vi "Facade.vi"(0 "Data In":T4, 2 "Display State In":T2, 3 "Container State":T3) -> (6 "Data Out":T4, 7 "Display State Out":T2, 8 "Action":T1)   [LabVIEW 2020, in "AM.xctl"]
uses:
  AM.xctl
  Data.vi
  Classes/Modulations/AM/AM.lvclass
  D:/Development/epl-vi-lib/Koop/KObject Class/KObject.lvclass
  <vilib>/_xctls/Container State.ctl
  State.vi
  <vilib>/_xctls/Action.ctl
  SAM/SAM.xctl
  Classes/Modulations/SAM/SAM.lvclass
  D:/Development/epl-vi-lib/Signal Synthesis VIs/4th Generation/Classes/Modulations/AM/AM.lvclass
  Classes/Modulations/AM/AM.lvclass/AM.ctl
  Classes/Modulations/AM/Write Depth (0-1).vi
  Classes/Modulations/AM/Write Correct level .vi
  Classes/Modulations/AM/Read Depth (0-1).vi
  Classes/Modulations/AM/Read Correct level .vi
  <vilib>/_xctls/XControlSupport.lvlib
  Koop/KObject Class/KObject.lvclass
panel:
  in  "Apply level correction":bool
  in  "Depth (0-1)":dbl min=0.0 max=1.0
  in  "Tabs":enum32{"OFF", "SAM"}(tab)
  in  "SAM":refnum<class "SAM.lvclass">(xcontrol)
  in  "Shape":u16(ring) items=["OFF", "SAM"]
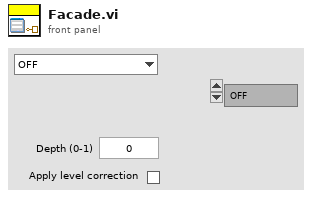
[diagram p1: front panel]
types:
  T1 = typedef "XControlSupport.lvlib/Action.ctl" = cluster{"Data Changed?":bool, "State Changed?":bool, "Action Name":string}
  T2 = typedef "AM.xctl/State.vi" = cluster{"Numeric":dbl}
  T3 = typedef "XControlSupport.lvlib/Container State.ctl" = cluster{"Indicator?":bool, "Run Mode?":bool, " Refnum":refnum<vi>}
  T4 = typedef "AM.xctl/Data.vi" = refnum<class "AM.lvclass">
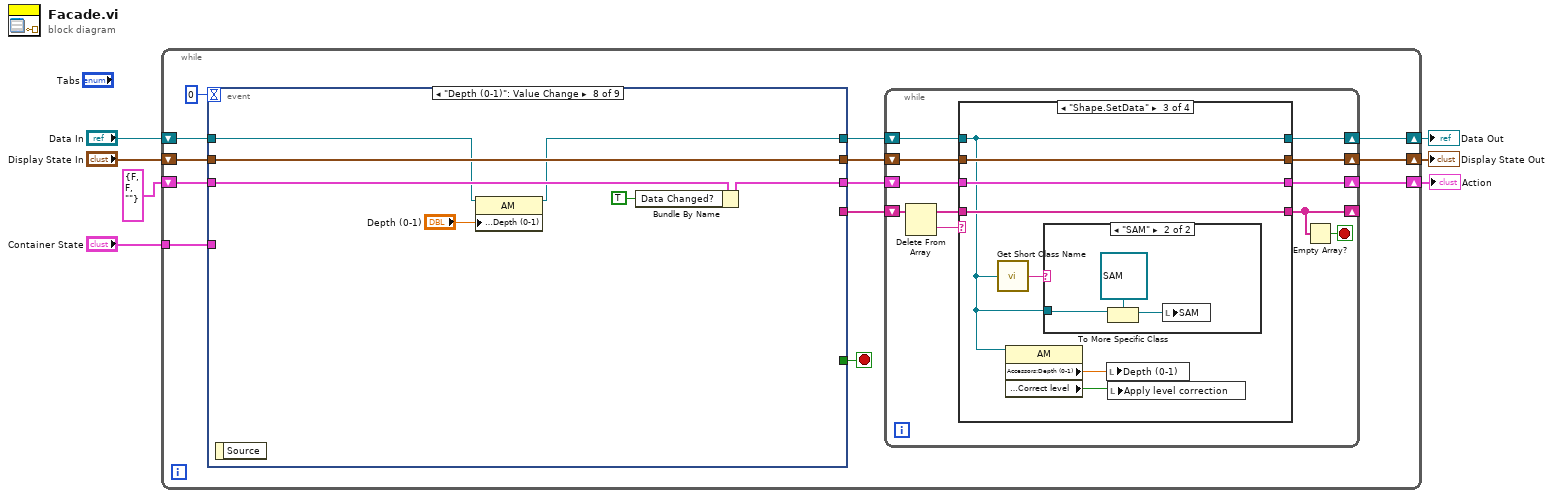
[diagram p0: block diagram]
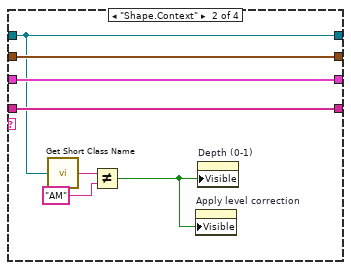
[diagram p3: hidden frame]
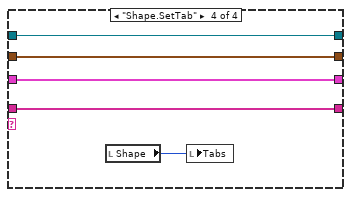
[diagram p5: hidden frame]
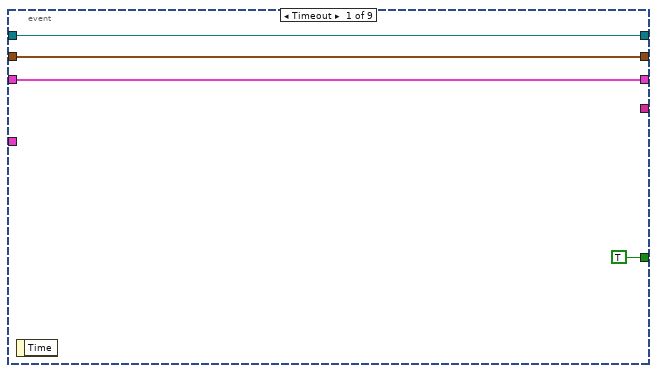
[diagram p6: hidden frame]
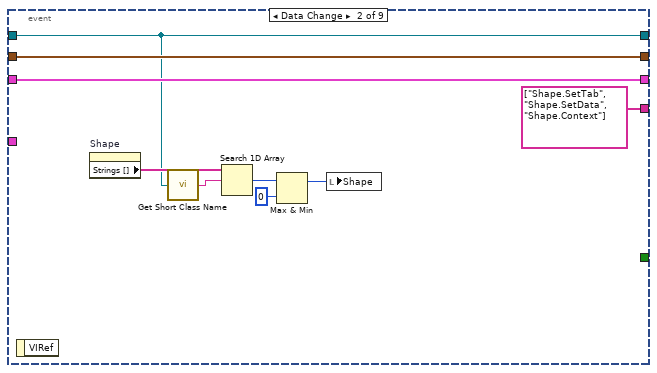
[diagram p7: hidden frame]
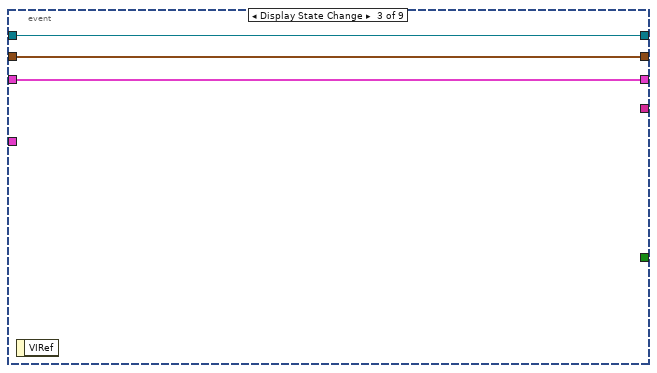
[diagram p8: hidden frame]
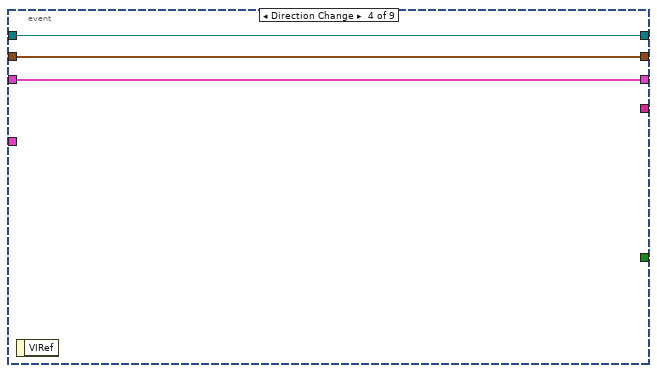
[diagram p9: hidden frame]
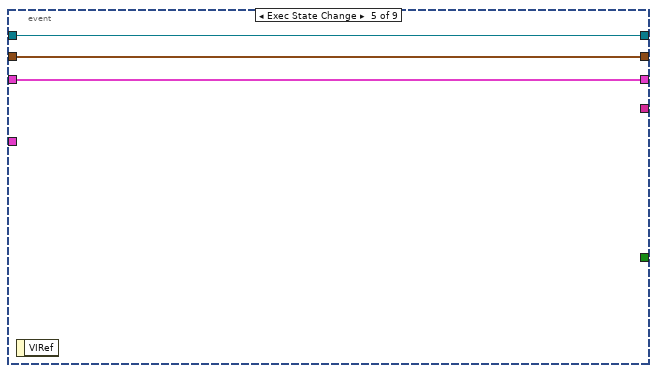
[diagram p10: hidden frame]
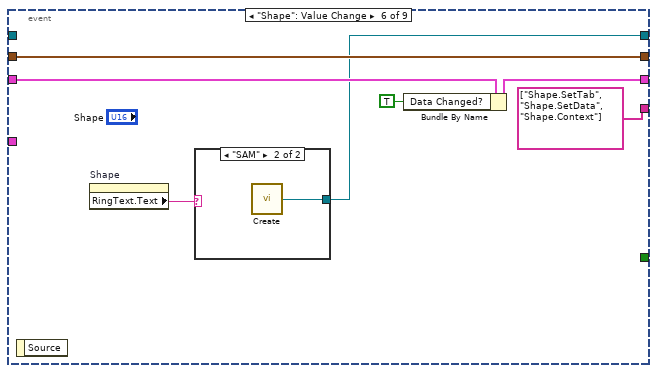
[diagram p11: hidden frame]
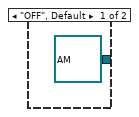
[diagram p12: hidden frame]
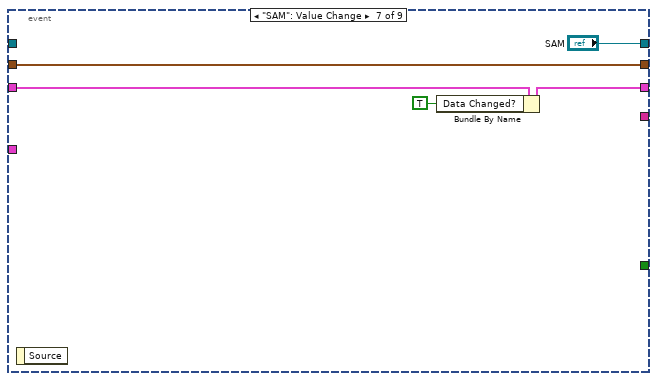
[diagram p13: hidden frame]
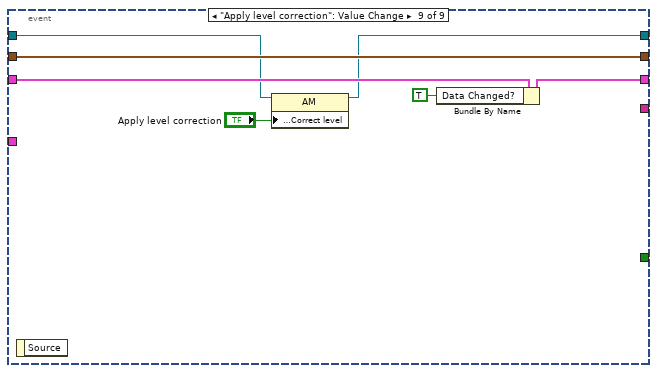
[diagram p14: hidden frame]
diagram:
  n1 = while {
    shift-right: [w11] -> w4
    shift-left: "Display State In" -> [w20]
    tunnel: "Container State" -> [w17]
    shift-right: [w13] -> w7
    shift-left: "Data In" -> [w16]
    shift-right: [w9] -> w2
    shift-left: T1 {"Data Changed?"=FALSE, "State Changed?"=FALSE, "Action Name"=""} ("Action") -> [w15]
    stop <- w19 stop-if-true
    n2 = event shown="[7] \"Depth (0-1)\": Value Change" {
      selector: _ -> [_ _ _ _ _ _ _ _ _]
      dyn-events: _ -> [_ _ _ _ _ _ _ _ _]
      timeout: 0 -> [_ _ _ _ _ _ _ _ _]
      tunnel: w20 -> [w59 w70 w73 w76 w79 w86 w93 w100 w107]
      tunnel: [w59 w70 w73 w76 w79 w86 w93 w100 w107] -> w12
      tunnel: [TRUE _ _ _ _ _ _ _ _] -> w19
      tunnel: w17 -> [_ _ _ _ _ _ _ _ _]
      tunnel: w16 -> [w58 w62 w72 w75 w77 _ _ w96 w103]
      tunnel: [w58 w62 w72 w75 w77 w82 "SAM" w95 w102] -> w14
      tunnel: [w60 w69 w71 w74 w78 w81 w90 w98 w105] -> w10
      tunnel: w15 -> [w60 w69 w71 w74 w78 w85 w92 w99 w106]
      tunnel: [_ string[] ["Shape.SetTab", "Shape.SetData", "Shape.Context"] _ _ _ string[] ["Shape.SetTab", "Shape.SetData", "Shape.Context"] _ _ _] -> w8
      event Timeout {
        n3 = event-data() -> ()  [unwired: 1 in, 1 out]
      }
      event Data Change {
        n4 = event-data() -> ()  [unwired: 1 in, 1 out]
        n5 = property on="Shape" class="Ring (strict)"() -> ("Strings []"=w65:string[])  [unwired: 2 in, 2 out]
        n6 = call "Get Short Class Name.vi"("KObject in"=w62) -> ("Class"=w66:string)  [unwired: 4 in]
        n7 = Search 1D Array(1D array=w65, element=w66) -> (index of element=w67:i32)  [unwired: 1 in]
        n8 = Max & Min(x=w67, y=0) -> (max(x,y)=w64:i32)  [unwired: 1 out]
        n9 = local write "Shape"(w64) -> ()
      }
      event Display State Change {
        n10 = event-data() -> ()  [unwired: 1 in, 1 out]
      }
      event Direction Change {
        n11 = event-data() -> ()  [unwired: 1 in, 1 out]
      }
      event Exec State Change {
        n12 = event-data() -> ()  [unwired: 1 in, 1 out]
      }
      event "Shape": Value Change {
        n13 = event-data() -> ()  [unwired: 1 in, 1 out]
        n14 = property on="Shape" class="Ring (strict)"() -> ("RingText.Text"=w83:string)  [unwired: 2 in, 2 out]
        n15 = case shown="\"SAM\"" w83 {
          tunnel: [refnum<class "AM.lvclass"> refnum ("AM") w88] -> w82
          frame "OFF", Default {
          }
          frame "SAM" {
            n16 = call "Create.vi"() -> ("SAM"=w88:refnum<class "SAM.lvclass">)  [unwired: 15 in]
          }
        }
        n17 = Bundle By Name(cluster=w85, "Data Changed?"=TRUE) -> (w81:T1)
      }
      event "SAM": Value Change {
        n18 = event-data() -> ()  [unwired: 1 in, 1 out]
        n19 = Bundle By Name(cluster=w92, "Data Changed?"=TRUE) -> (w90:T1)
      }
      event "Depth (0-1)": Value Change {
        n20 = event-data() -> ()  [unwired: 1 in, 1 out]
        n21 = property class="AM"(reference=w96, "Accessors:Depth (0-1)"="Depth (0-1)") -> (reference out=w95:T4)  [unwired: 1 in, 1 out]
        n22 = Bundle By Name(cluster=w99, "Data Changed?"=TRUE) -> (w98:T1)
      }
      event "Apply level correction": Value Change {
        n23 = event-data() -> ()  [unwired: 1 in, 1 out]
        n24 = property class="AM"(reference=w103, "Accessors:Correct level "="Apply level correction") -> (reference out=w102:T4)  [unwired: 1 in, 1 out]
        n25 = Bundle By Name(cluster=w106, "Data Changed?"=TRUE) -> (w105:T1)
      }
    }
    n26 = while {
      shift-right: [w28] -> _
      shift-left: w8 -> [w31]
      shift-right: [w23] -> w13
      shift-left: w14 -> [w26]
      shift-right: [w22] -> w11
      shift-left: w12 -> [w25]
      shift-right: [w21] -> w9
      shift-left: w10 -> [w24]
      stop <- w27 stop-if-true
      n27 = Delete From Array(array=w31) -> (deleted portion=w29:string, array with subset deleted=w30:string[])  [unwired: 2 in]
      n28 = case shown="\"Shape.SetData\"" w29 {
        tunnel: w30 -> [w35 w42 w49 w57]
        tunnel: [w35 w42 w49 w57] -> w28
        tunnel: w26 -> [w34 w39 w43 w56]
        tunnel: w25 -> [w33 w41 w48 w55]
        tunnel: w24 -> [w32 w40 w47 w54]
        tunnel: [w34 w39 w43 w56] -> w23
        tunnel: [w33 w41 w48 w55] -> w22
        tunnel: [w32 w40 w47 w54] -> w21
        frame "", Default {
        }
        frame "Shape.Context" {
          n29 = call "Get Short Class Name.vi"("KObject in"=w39) -> ("Class"=w38:string)  [unwired: 4 in]
          n30 = Not Equal?(x=w38, y="AM") -> (x != y?=w36:bool)
          n31 = property on="Apply level correction" class="Bool (strict)"("Visible"=w36) -> ()  [unwired: 2 in, 2 out]
          n32 = property on="Depth (0-1)" class="DigNum (strict)"("Visible"=w36) -> ()  [unwired: 2 in, 2 out]
        }
        frame "Shape.SetData" {
          n33 = call "Get Short Class Name.vi"("KObject in"=w43) -> ("Class"=w46:string)  [unwired: 4 in]
          n34 = property class="AM"(reference=w43) -> ("Accessors:Depth (0-1)"=w44:dbl, "Accessors:Correct level "=w45:bool)  [unwired: 1 in, 2 out]
          n35 = case shown="\"SAM\"" w46 {
            tunnel: w43 -> [_ w52]
            frame "OFF", Default {
            }
            frame "SAM" {
              n36 = To More Specific Class(target class=refnum<class "SAM.lvclass"> refnum ("SAM"), reference=w52) -> (specific class reference=w51:refnum<class "SAM.lvclass">)  [unwired: 1 in, 1 out]
              n37 = local write "SAM"(w51) -> ()
            }
          }
          n38 = local write "Depth (0-1)"(w44) -> ()
          n39 = local write "Apply level correction"(w45) -> ()
        }
        frame "Shape.SetTab" {
          n40 = local read "Shape"() -> (w53:u16)
          n41 = local write "Tabs"(w53) -> ()
        }
      }
      n42 = Empty Array?(array=w28) -> (empty?=w27:bool)
    }
  }
  "Display State Out" <- w4
  "Data Out" <- w7
  "Action" <- w2
